vi "Acquire Voltage.vi"(8 "error in (no error)":errorcluster, 11 "Analog Input in":refnum<class "Analog Input.lvclass">) -> (0 "error out":errorcluster, 3 "Analog Input out":refnum<class "Analog Input.lvclass">)   [LabVIEW 2021, in "Analog Input.lvclass"]
uses:
  Analog Input.lvclass
  C:/Program Files/National Instruments/LabVIEW 2021/vi.lib/ActorFramework/Actor/Actor.lvclass
  <vilib>/ActorFramework/Actor/Actor.lvclass/Actor.ctl
  <vilib>/ActorFramework/Message Enqueuer/Message Enqueuer.lvclass/Message Enqueuer.ctl
  Analog Input.lvclass/Analog Input.ctl
  Analog Input Interface Messages/Analog Input Interface Messages Messages/Analog Input Voltages Msg/Analog Input Voltages Msg.lvclass/Analog Input Voltages Msg.ctl
  <vilib>/DAQmx/read.llb/DAQmx Read (Analog 1D Wfm NChan NSamp).vi
  <vilib>/ActorFramework/Message Enqueuer/Init from Existing Queue.vi
  <vilib>/ActorFramework/Message Enqueuer/Enqueue.vi
  Analog Input Messages/Acquire Voltage Msg/Acquire Voltage Msg.lvclass
  C:/Program Files/National Instruments/LabVIEW 2021/vi.lib/ActorFramework/Message/Message.lvclass
  Analog Input Interface Messages/Analog Input Interface Messages Messages/Analog Input Voltages Msg/Analog Input Voltages Msg.lvclass
  <vilib>/ActorFramework/Message Priority Queue/Priority Enqueue.vi
  <vilib>/DAQmx/miscellaneous.llb/DAQmx Fill In Error Info.vi
  <vilib>/ActorFramework/Message Enqueuer/Message Enqueuer.lvclass
  <vilib>/ActorFramework/Actor/Actor.lvclass
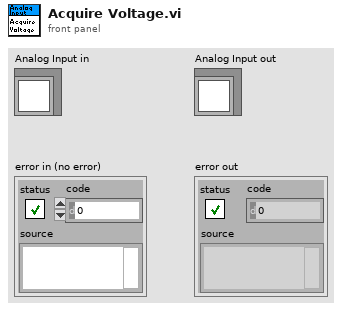
[diagram p1: front panel]
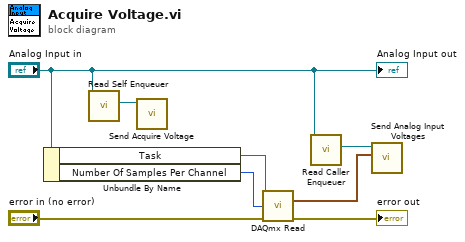
[diagram p0: block diagram]
diagram:
  n1 = Unbundle By Name("Analog Input in") -> ("Task"=w7:refnum<k21>, "Number Of Samples Per Channel"=w8:i32)
  n2 = call <vilib>:"Read Self Enqueuer.vi"("Actor"="Analog Input in") -> ("Self Enqueuer"=w5:refnum<class "Message Enqueuer.lvclass">)  [unwired: 10 in]
  n3 = call "Send Acquire Voltage.vi"("Message Enqueuer"=w5) -> ()  [unwired: 9 in, 2 out]
  n4 = call-poly <vilib>:"DAQmx Read.vi"("task/channels in"=w7, "number of samples per channel"=w8, "error in"="error in (no error)") -> ("data"=w4:waveform(dbl)[], "error out"=→"error out":errorcluster)  [unwired: 10 in, 1 out]
  n5 = call <vilib>:"Read Caller Enqueuer.vi"("Actor"="Analog Input in") -> ("Caller Enqueuer"=w6:refnum<class "Message Enqueuer.lvclass">)  [unwired: 10 in]
  n6 = call "Send Analog Input Voltages.vi"("Analog Input Voltages"=w4, "Message Enqueuer"=w6) -> ()  [unwired: 8 in, 2 out]
  "Analog Input out" <- "Analog Input in"
